vi "process network stream messages.vi"(11 "Cluster":cluster{"message":string, "data":variant}) -> (2 "type":string, 3 "data":T1)   [LabVIEW 2018]
uses:
  RT/Type Defs/generic incident.ctl
panel:
  out "error out":errorcluster
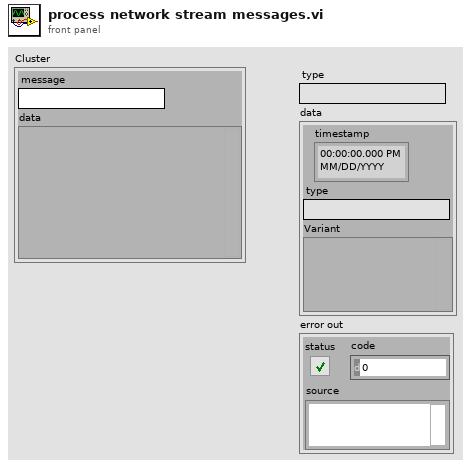
[diagram p1: front panel]
types:
  T1 = typedef "generic incident.ctl" = cluster{"timestamp":timestamp, "type":string, "Variant":variant}
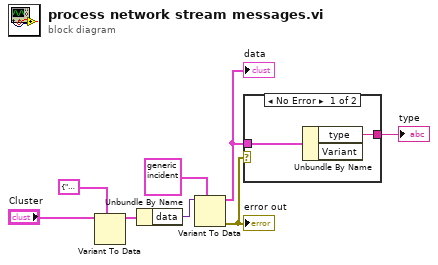
[diagram p0: block diagram]
diagram:
  n1 = Variant To Data(type=cluster{"message":string, "data":variant} {"message"="", "data"=variant}, Variant="Cluster") -> (data=w6:cluster{"message":string, "data":variant})  [unwired: 1 in, 1 out]
  n2 = Unbundle By Name(w6) -> ("data"=w7:variant)
  n3 = Variant To Data(type=T1 {"timestamp"=timestamp(0 s since 1904-01-01), "type"="", "Variant"=variant} ("incident cluster"), Variant=w7) -> (data=w2:T1, error out=w1:errorcluster)  [unwired: 1 in]
  "data" <- w2
  "error out" <- w1
  n4 = case shown="No Error" w1 {
    tunnel: [w10 _] -> w4
    tunnel: w2 -> [w9 _]
    frame No Error {
      n5 = Unbundle By Name(w9) -> ("type"=w10:string)  [unwired: 1 out]
    }
    frame Error {
    }
  }
  "type" <- w4
